vi "Load Into Sub Panel.vi"(8 "error in (no error)":errorcluster, 10 "VI for SubPanel":refnum<vi>, 11 "Air Cooler Application in":refnum<class "Air Cooler Application.lvclass">) -> (0 "error out":errorcluster, 3 "Air Cooler Application out":refnum<class "Air Cooler Application.lvclass">)   [LabVIEW 2025, in "Air Cooler Application.lvlib" / "Air Cooler Application.lvclass"]
uses:
  Air Cooler Application.lvclass
  Air Cooler Application.lvclass/Air Cooler Application.ctl
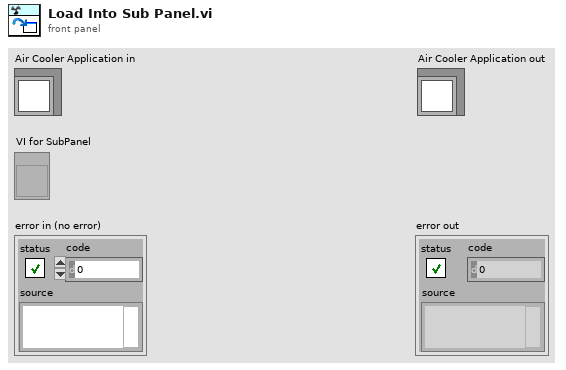
[diagram p1: front panel]
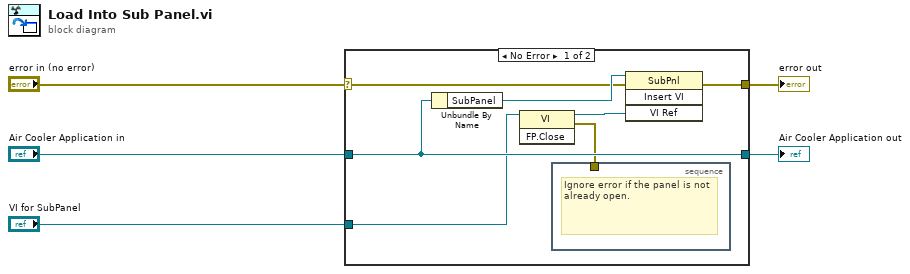
[diagram p0: block diagram]
diagram:
  n1 = case shown="No Error" "error in (no error)" {
    selector: "error in (no error)" -> [w10 w14]
    tunnel: [w9 w14] -> w4
    tunnel: [w12 w13] -> w2
    tunnel: "Air Cooler Application in" -> [w12 w13]
    tunnel: "VI for SubPanel" -> [w8 _]
    frame No Error {
      n2 = Unbundle By Name(w12) -> ("SubPanel"=w11:refnum<vi>)
      n3 = invoke class="VI" method="FP.Close"(reference=w8) -> (reference out=w7:refnum<vi>, error out=w6:errorcluster)  [unwired: 2 in, 1 out]
      n4 = stacked-sequence {
        tunnel: w6 -> [_]
        frame #0 {
          # "Ignore error if the panel is not already open."
        }
      }
      n5 = invoke on="Invoke Node" class="SubPnl" method="Insert VI"(reference=w11, error in=w10, "VI Ref"=w7) -> (error out=w9:errorcluster)  [unwired: 1 in, 3 out]
    }
    frame Error {
    }
  }
  "error out" <- w4
  "Air Cooler Application out" <- w2
